vi "Threshold FPGA.vi"() -> ()   [LabVIEW 2010]
uses:
  <vilib>/eio/EIONode/EIONode.xnode
  <vilib>/rvi/eio/nirviEIOImplementation/nirviEIOImplementation.xnode
  <vilib>/rvi/eio/common/nirviEmuClasses.ctl
  <vilib>/rvi/eio/common/nirviEmuTemplateMethod_noerrors.vi
panel:
  in  "Stop FPGA":bool
  out "Threshold Exceeded":bool
  in  "Threshold (binary)":i16
  out "AI0 (binary)":i16
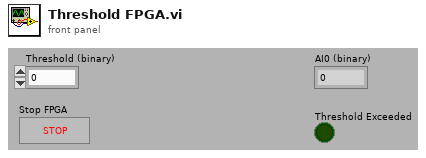
[diagram p1: front panel]
types:
  T1 = typedef "nirviEmuClasses.ctl" = enum16{"IO Read", "IO Write", "Method", "Property Read", "Property Write"}
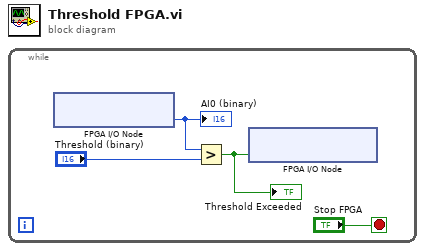
[diagram p0: block diagram]
diagram:
  n1 = while {
    stop <- "Stop FPGA" stop-if-true
    n2 = xnode "FPGA I/O Node"() -> ("Connector0/AI0"=w4:i16)  [unwired: 1 in, 1 out]
    "AI0 (binary)" <- w4
    n3 = Greater?(x=w4, y="Threshold (binary)") -> (0:w3:bool)
    "Threshold Exceeded" <- w3
    n4 = xnode "FPGA I/O Node"("Connector0/DIO0"=w3) -> ()  [unwired: 1 in, 1 out]
  }
